vi "State_Machine.vi"(8 "error in (no error)":errorcluster caption="entrée d'erreur (pas d'erreur)", 11 "Wait_CloseFixture en entrée":refnum<class "Wait_CloseFixture.lvclass">) -> (0 "error out":errorcluster caption="sortie d'erreur", 2 "Json_String":string, 3 "Wait_CloseFixture en sortie":refnum<class "Wait_CloseFixture.lvclass">)   [LabVIEW 2020, in "Library Test.lvlib" / "Wait_CloseFixture.lvclass"]
uses:
  Wait_CloseFixture.lvclass
  C:/Users/ngarcin/OneDrive - Altyor/Standard TB/Class/Test/Test (Default)/Test (Default).lvclass
  Instrument/Instrument (Default)/Class Instrument (Default).lvclass
  Popup/Class Popup WaitDIO/Class Popup WaitDIO.lvclass
  C:/Users/ngarcin/OneDrive - Altyor/Standard TB/Class/Popup/Class Popup Operator_Validation/Class Popup Operator_Validation (Default)/Class Popup Operator_Validation (Virtual).lvclass
  C:/Users/ngarcin/OneDrive - Altyor/Standard TB/Class/Popup/Class Popup (Main)/Class Popup (Main).lvclass
  Wait_CloseFixture.lvclass/Wait_CloseFixture.ctl
  Commun VI/Library Commun.lvlib
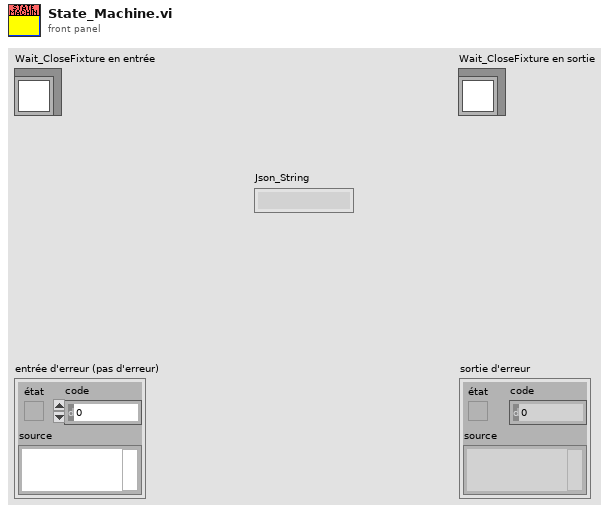
[diagram p1: front panel]
types:
  T1 = cluster{"Instrument DIO":refnum<class "Class Instrument (Default).lvclass">, "Valur for test":bool, "Timeout (ms)":u64}
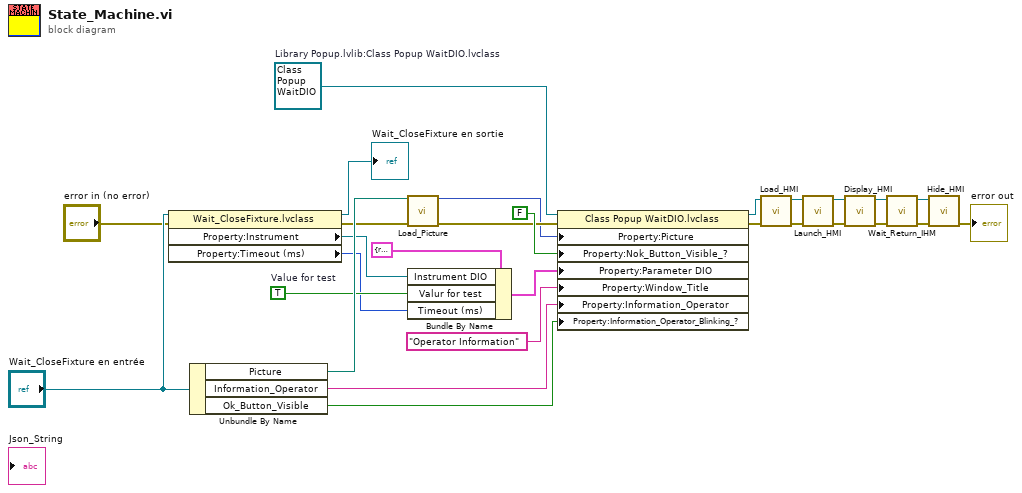
[diagram p0: block diagram]
diagram:
  w9 = refnum<class "Class Popup WaitDIO.lvclass"> refnum  # Library Popup.lvlib:Class Popup WaitDIO.lvclass
  w13 = TRUE  # Value for test
  n1 = property class="Wait_CloseFixture.lvclass"(reference="Wait_CloseFixture en entrée", error in="error in (no error)") -> (reference out=→"Wait_CloseFixture en sortie":refnum<class "Wait_CloseFixture.lvclass">, error out=w2:errorcluster, "Property:Instrument"=w4:refnum<class "Class Instrument (Default).lvclass">, "Property:Timeout (ms)"=w10:u64)
  n2 = Unbundle By Name("Wait_CloseFixture en entrée") -> ("Picture"=w20:path, "Information_Operator"=w23:string, "Ok_Button_Visible"=w22:bool)
  n3 = call "Load_Picture.vi"("Chemin In"=w20, "error in (no error)"=w2) -> ("Img Out"=w19:picture, "error out"=w21:errorcluster)  [unwired: 11 in, 1 out]
  n4 = Bundle By Name(cluster=T1 {"Instrument DIO"=refnum, "Valur for test"=FALSE, "Timeout (ms)"=0}, "Instrument DIO"=w4, "Valur for test"=w13, "Timeout (ms)"=w10) -> (w1:T1)
  n5 = property class="Class Popup WaitDIO.lvclass"(reference=w9, error in=w21, "Property:Picture"=w19, "Property:Nok_Button_Visible_?"=FALSE ("Nok_Button_Visible_?"), "Property:Parameter DIO"=w1, "Property:Window_Title"="Operator Information" ("Window_Title"), "Property:Information_Operator"=w23, "Property:Information_Operator_Blinking_?"=w22) -> (reference out=w27:refnum<class "Class Popup WaitDIO.lvclass">, error out=w26:errorcluster)
  n6 = call-dynamic "Load_HMI.vi"("error in (no error)"=w26, "Class Popup (Default) en entrée"=w27) -> ("error out"=w16:errorcluster, "Class Popup (Default) en sortie"=w17:refnum<class "Class Popup WaitDIO.lvclass">)  [unwired: 8 in]
  n7 = call-dynamic "Launch_HMI.vi"("error in (no error)"=w16, "Class Popup (Default) en entrée"=w17) -> ("error out"=w28:errorcluster, "Class Popup (Default) en sortie"=w18:refnum<class "Class Popup WaitDIO.lvclass">)  [unwired: 8 in]
  n8 = call-dynamic "Display_HMI.vi"("error in (no error)"=w28, "Class Popup (Default) en entrée"=w18) -> ("error out"=w8:errorcluster, "Class Popup (Default) en sortie"=w5:refnum<class "Class Popup WaitDIO.lvclass">)  [unwired: 8 in]
  n9 = call-dynamic "Wait_Return_IHM.vi"("error in (no error)"=w8, "Class Popup (Default) en entrée"=w5) -> ("error out"=w7:errorcluster, "Class Popup (Default) en sortie"=w6:refnum<class "Class Popup WaitDIO.lvclass">)  [unwired: 8 in]
  n10 = call-dynamic "Hide_HMI.vi"("error in (no error)"=w7, "Class Popup (Default) en entrée"=w6) -> ("error out"=→"error out":errorcluster)  [unwired: 8 in, 1 out]
